vi "Menu.Sequence.Load.vi"(8 "error in (no error)":errorcluster, 9 "MenuRef":refnum<k9>, 10 "Coords":T1, 11 "Cluster in":T2) -> (0 "error out":errorcluster, 3 "Cluster out":T2)   [LabVIEW 2013]
uses:
  Types/StateVariables.ctl
  Types/ChannelProperties.ctl
  <vilib>/Utility/miscctls.llb/LVPoint32TypeDef.ctl
  Constants.vi
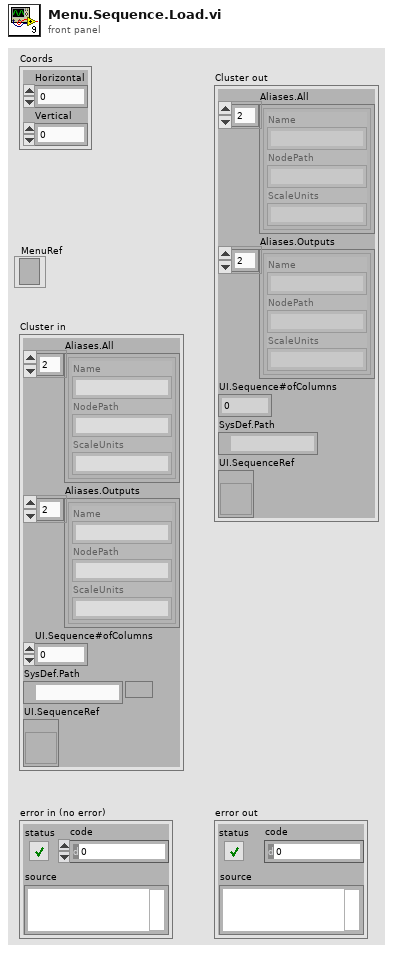
[diagram p1: front panel]
types:
  T1 = typedef "LVPoint32TypeDef.ctl" = cluster{"Horizontal":i32, "Vertical":i32}
  T2 = typedef "StateVariables.ctl" = cluster{"Aliases.All":T3[], "Aliases.Outputs":T3[], "UI.Sequence#ofColumns":i32, "SysDef.Path":path, "UI.SequenceRef":refnum<vi>}
  T3 = typedef "ChannelProperties.ctl" = cluster{"Name":string, "NodePath":string, "ScaleUnits":string}
  T4 = typedef "LVRowAndColumnTypeDef.ctl" = cluster{"Row":i32, "Column":i32}
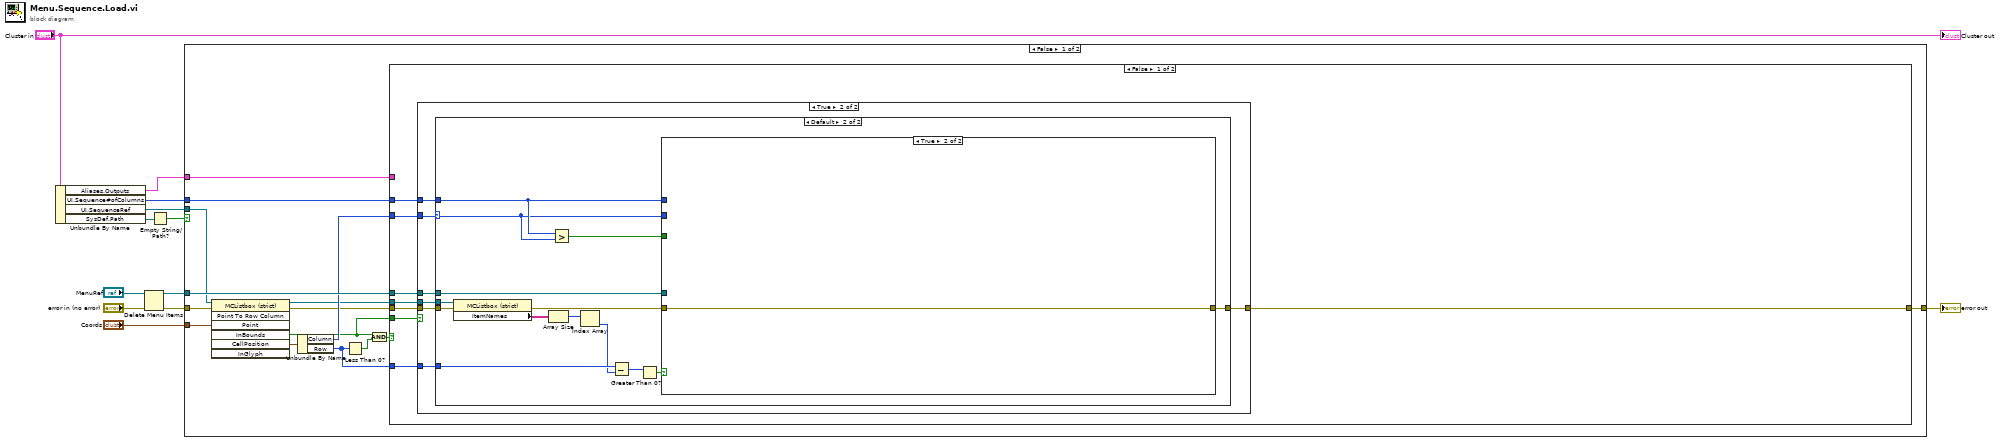
[diagram p0: block diagram]
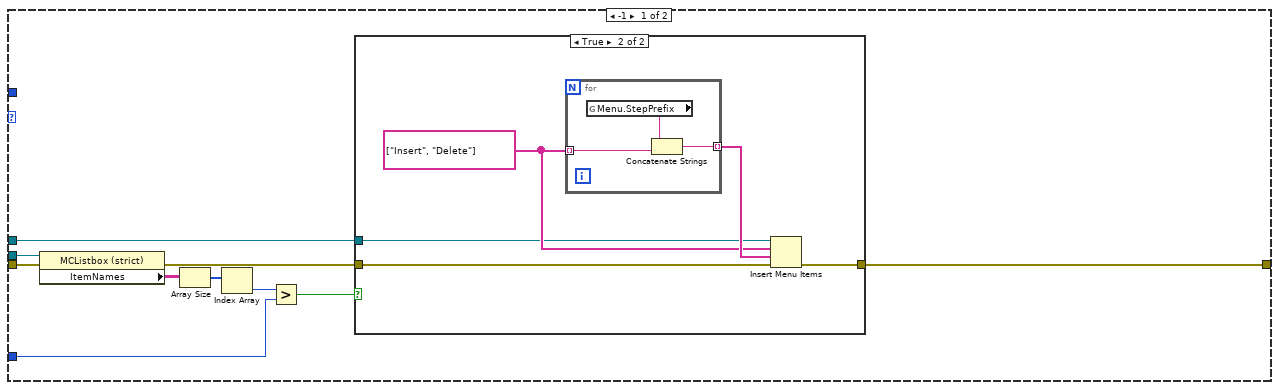
[diagram p3: hidden frame]
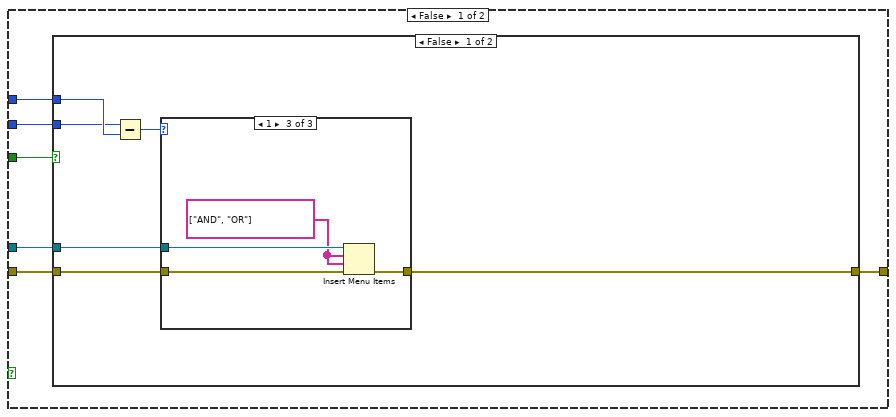
[diagram p5: hidden frame]
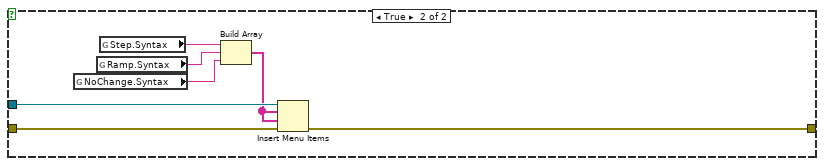
[diagram p8: hidden frame]
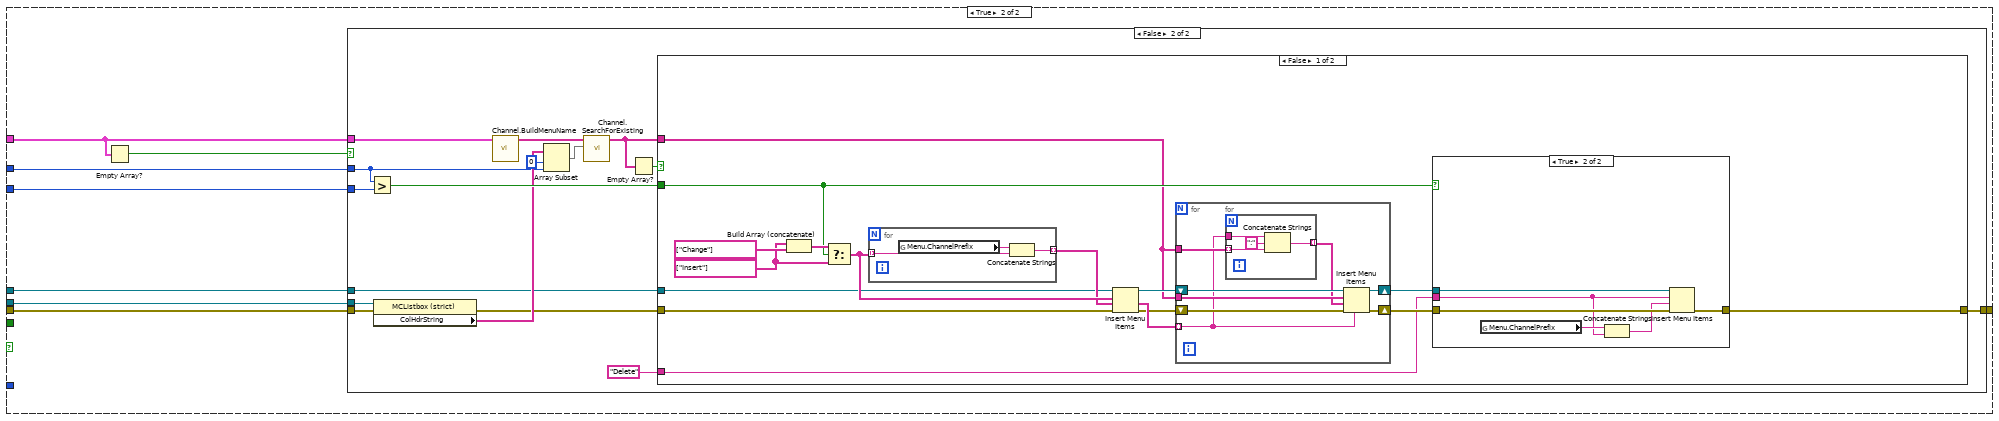
[diagram p9: hidden frame]
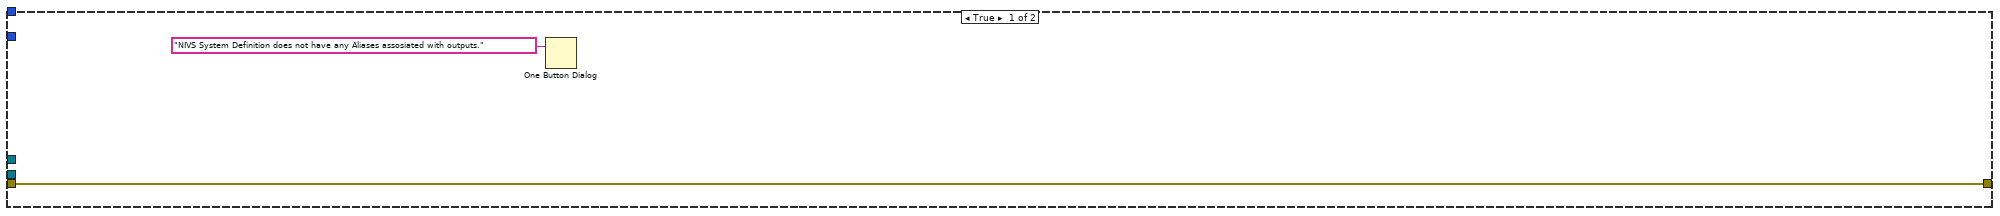
[diagram p10: hidden frame]
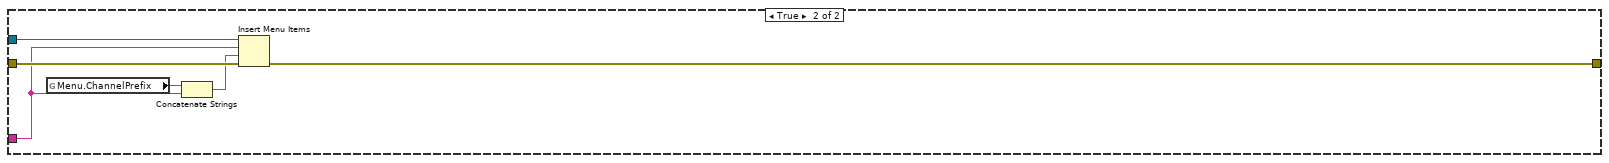
[diagram p12: hidden frame]
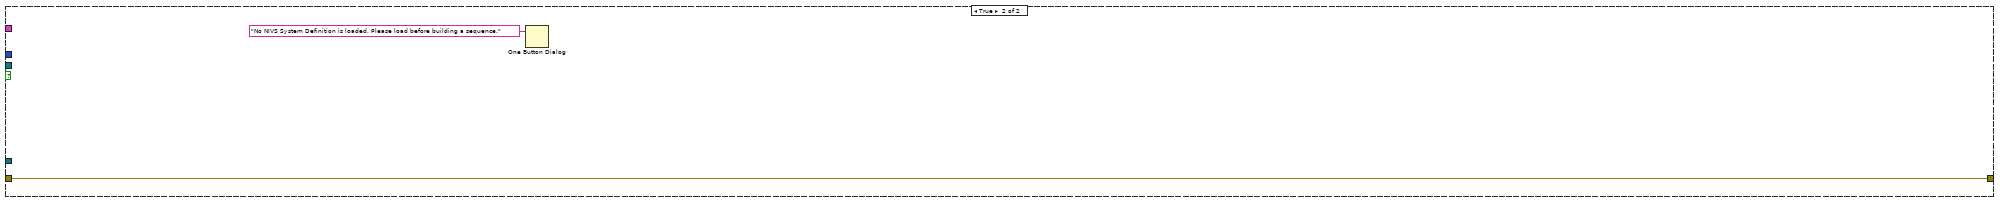
[diagram p13: hidden frame]
diagram:
  n1 = Unbundle By Name("Cluster in") -> ("Aliases.Outputs"=w8:T3[], "UI.Sequence#ofColumns"=w11:i32, "UI.SequenceRef"=w9:refnum<vi>, "SysDef.Path"=w6:path)
  n2 = Delete Menu Items(6:"error in (no error)", 9:"MenuRef") -> (0:w3:errorcluster, 3:w1:refnum<k9>)  [unwired: 2 in]
  n3 = Empty String/Path?(string/path=w6) -> (empty?=w5:bool)
  n4 = case shown="False" w5 {
    tunnel: [w27 w173] -> w12
    tunnel: w1 -> [w26 _]
    tunnel: w11 -> [w25 _]
    tunnel: "Coords" -> [w20 _]
    tunnel: w9 -> [w19 _]
    tunnel: w3 -> [w18 w173]
    tunnel: w8 -> [w15 _]
    frame False {
      n5 = invoke class="MCListbox (strict)" method="Point To Row Column"(reference=w19, error in=w18, "Point"=w20) -> (reference out=w16:refnum<vi>, error out=w17:errorcluster, "InBounds"=w14:bool, "CellPosition"=w21:T4)  [unwired: 4 in, 3 out]
      n6 = Unbundle By Name(w21) -> ("Column"=w24:i32, "Row"=w13:i32)
      n7 = Less Than 0?(x=w13) -> (x < 0?=w22:bool)
      n8 = And(x=w14, y=w22) -> (x .and. y?=w23:bool)
      n9 = case shown="False" w23 {
        tunnel: w24 -> [w30 w110]
        tunnel: w25 -> [w31 w108]
        tunnel: w26 -> [w29 w105]
        tunnel: w17 -> [w34 w106]
        tunnel: [w28 w107] -> w27
        tunnel: w16 -> [w33 w109]
        tunnel: w15 -> [_ w104]
        tunnel: w14 -> [w35 _]
        tunnel: w13 -> [w32 _]
        frame False {
          n10 = case shown="True" w35 {
            tunnel: w34 -> [w36 w42]
            tunnel: w33 -> [_ w43]
            tunnel: w32 -> [_ w41]
            tunnel: w31 -> [_ w40]
            tunnel: w30 -> [_ w39]
            tunnel: w29 -> [_ w38]
            tunnel: [w36 w37] -> w28
            frame False {
            }
            frame True {
              n11 = case shown="Default" w39 {
                selector: w39 -> [_ w66]
                tunnel: w43 -> [w49 w76]
                tunnel: w42 -> [w51 w75]
                tunnel: w41 -> [w46 w72]
                tunnel: w40 -> [_ w67]
                tunnel: w38 -> [w52 w68]
                tunnel: [w53 w64] -> w37
                frame -1 {
                  n12 = property class="MCListbox (strict)"(reference=w49, error in=w51) -> (error out=w50:errorcluster, "ItemNames"=w47:string[][])  [unwired: 1 out]
                  n13 = Array Size(array=w47) -> (size(s)=w48:i32[])
                  n14 = Index Array(array=w48) -> (element=w45:i32)  [unwired: 1 in]
                  n15 = Greater?(x=w45, y=w46) -> (0:w44:bool)
                  n16 = case shown="True" w44 {
                    tunnel: [w54 w59] -> w53
                    tunnel: w52 -> [_ w56]
                    tunnel: w50 -> [w54 w55]
                    frame False {
                    }
                    frame True {
                      w57 = string[] ["Insert", "Delete"] ("item names")
                      n17 = for {
                        tunnel: [w61] -> w58 mode=indexing
                        tunnel: w57 -> [w62] mode=indexing
                        n18 = global read "Constants.vi" "Menu.StepPrefix"() -> (w60:string)
                        n19 = Concatenate Strings(w60, w62) -> (w61:string)
                      }
                      n20 = Insert Menu Items(6:w55, 7:w58, 8:w57, 9:w56) -> (0:w59:errorcluster)  [unwired: 2 in, 2 out]
                    }
                  }
                }
                frame Default {
                  n21 = property class="MCListbox (strict)"(reference=w76, error in=w75) -> (error out=w70:errorcluster, "ItemNames"=w74:string[][])  [unwired: 1 out]
                  n22 = Array Size(array=w74) -> (size(s)=w73:i32[])
                  n23 = Greater?(x=w67, y=w66) -> (0:w65:bool)
                  n24 = Index Array(array=w73) -> (element=w71:i32)  [unwired: 1 in]
                  n25 = Subtract(x=w72, y=w71) -> (x-y=w63:i32)
                  n26 = Greater Than 0?(x=w63) -> (x > 0?=w69:bool)
                  n27 = case shown="True" w69 {
                    tunnel: w70 -> [w82 w102]
                    tunnel: w67 -> [w79 _]
                    tunnel: w66 -> [w78 _]
                    tunnel: w68 -> [w81 _]
                    tunnel: w65 -> [w80 _]
                    tunnel: [w77 w102] -> w64
                    frame False {
                      n28 = case shown="False" w80 {
                        tunnel: w82 -> [w84 w101]
                        tunnel: w81 -> [w85 w99]
                        tunnel: w79 -> [w88 _]
                        tunnel: w78 -> [w87 _]
                        tunnel: [w83 w100] -> w77
                        frame False {
                          n29 = Subtract(x=w87, y=w88) -> (x-y=w86:i32)
                          n30 = case shown="1" w86 {
                            tunnel: w85 -> [_ _ w94]
                            tunnel: w84 -> [w89 w90 w93]
                            tunnel: [w89 w90 w91] -> w83
                            frame Default {
                            }
                            frame 0 {
                            }
                            frame 1 {
                              w92 = string[] ["AND", "OR"] ("item names")
                              n31 = Insert Menu Items(6:w93, 7:w92, 8:w92, 9:w94) -> (0:w91:errorcluster)  [unwired: 2 in, 2 out]
                            }
                          }
                        }
                        frame True {
                          n32 = global read "Constants.vi" "NoChange.Syntax"() -> (w95:string)
                          n33 = global read "Constants.vi" "Ramp.Syntax"() -> (w97:string)
                          n34 = global read "Constants.vi" "Step.Syntax"() -> (w98:string)
                          n35 = Build Array(w98, w97, w95) -> (w96:string[])
                          n36 = Insert Menu Items(6:w101, 7:w96, 8:w96, 9:w99) -> (0:w100:errorcluster)  [unwired: 2 in, 2 out]
                        }
                      }
                    }
                    frame True {
                    }
                  }
                }
              }
            }
          }
        }
        frame True {
          n37 = Empty Array?(array=w104) -> (empty?=w103:bool)
          n38 = case shown="False" w103 {
            tunnel: w110 -> [_ w128]
            tunnel: w109 -> [_ w126]
            tunnel: w108 -> [_ w124]
            tunnel: [w112 w122] -> w107
            tunnel: w104 -> [_ w121]
            tunnel: w106 -> [w112 w117]
            tunnel: w105 -> [_ w118]
            frame True {
              n39 = One Button Dialog(message="NIVS System Definition does not have any Aliases assosiated with outputs.") -> ()  [unwired: 1 in, 1 out]
            }
            frame False {
              n40 = Greater?(x=w124, y=w128) -> (0:w127:bool)
              n41 = property class="MCListbox (strict)"(reference=w126, error in=w117) -> (error out=w116:errorcluster, "ColHdrString"=w125:string[])  [unwired: 1 out]
              n42 = call "Channel.BuildMenuName.vi"("Aliases.Outputs"=w121) -> ("Array"=w119:string[])  [unwired: 10 in]
              n43 = Array Subset(array=w125, index=0, length=w124) -> (w120:string[])
              n44 = call "Channel.SearchForExisting.vi"("Existing Channels"=w120, "All Channels"=w119) -> ("Array out"=w115:string[])  [unwired: 9 in]
              n45 = Empty Array?(array=w115) -> (empty?=w114:bool)
              n46 = case shown="False" w114 {
                tunnel: w127 -> [w130 _]
                tunnel: [w133 w171] -> w122
                tunnel: w118 -> [w137 w170]
                tunnel: w115 -> [w129 _]
                tunnel: w116 -> [w135 w172]
                tunnel: "Delete" ("string") -> [w131 w168]
                frame False {
                  w142 = string[] ["Insert"]
                  n47 = Build Array (concatenate)(w142, string[] ["Change"]) -> (w143:string[])
                  n48 = Select(t=w143, s=w130, f=w142) -> (s? t:f=w141:string[])
                  n49 = for {
                    tunnel: w141 -> [w166] mode=indexing
                    tunnel: [w165] -> w140 mode=indexing
                    n50 = global read "Constants.vi" "Menu.ChannelPrefix"() -> (w164:string)
                    n51 = Concatenate Strings(w164, w166) -> (w165:string)
                  }
                  n52 = Insert Menu Items(6:w135, 7:w140, 8:w141, 9:w137) -> (0:w136:errorcluster, 1:w138:string[], 3:w139:refnum<k9>)  [unwired: 2 in]
                  n53 = for {
                    tunnel: w138 -> [w153] mode=indexing
                    shift-right: [w158] -> w134
                    shift-left: w136 -> [w159]
                    tunnel: w129 -> [w156]
                    shift-right: [w155] -> w132
                    shift-left: w139 -> [w157]
                    tunnel: w129 -> [w154]
                    n54 = for {
                      tunnel: w154 -> [w163] mode=indexing
                      tunnel: w153 -> [w161]
                      tunnel: [w160] -> w152 mode=indexing
                      n55 = Concatenate Strings(w161, ":" ("string"), w163) -> (w160:string)
                    }
                    n56 = Insert Menu Items(5:w153, 6:w159, 7:w152, 8:w156, 9:w157) -> (0:w158:errorcluster, 3:w155:refnum<k9>)  [unwired: 1 in, 1 out]
                  }
                  n57 = case shown="True" w130 {
                    tunnel: w134 -> [w145 w151]
                    tunnel: [w145 w150] -> w133
                    tunnel: w132 -> [_ w149]
                    tunnel: w131 -> [_ w146]
                    frame False {
                    }
                    frame True {
                      n58 = global read "Constants.vi" "Menu.ChannelPrefix"() -> (w148:string)
                      n59 = Concatenate Strings(w148, w146) -> (w147:string)
                      n60 = Insert Menu Items(6:w151, 7:w147, 8:w146, 9:w149) -> (0:w150:errorcluster)  [unwired: 2 in, 2 out]
                    }
                  }
                }
                frame True {
                  n61 = global read "Constants.vi" "Menu.ChannelPrefix"() -> (w169:string)
                  n62 = Concatenate Strings(w169, w168) -> (w167:string)
                  n63 = Insert Menu Items(6:w172, 7:w167, 8:w168, 9:w170) -> (0:w171:errorcluster)  [unwired: 2 in, 2 out]
                }
              }
            }
          }
        }
      }
    }
    frame True {
      n64 = One Button Dialog(message="No NIVS System Definition is loaded. Please load before building a sequence.") -> ()  [unwired: 1 in, 1 out]
    }
  }
  "error out" <- w12
  "Cluster out" <- "Cluster in"
